vi "LV New.vi"(6 "Misc Project Files":path[](array[path]), 8 "error in (no error)":errorcluster, 9 "VI":path, 10 "Lvlib":path, 11 "Lvproj":path) -> (0 "error out":errorcluster)   [LabVIEW 2018, in "Pkg.lvlib"]
uses:
  Pkg.lvlib
  <vilib>/ErrorRing/Error Ring.xnode
  <vilib>/Utility/error.llb/Error Cluster From Error Code.vi
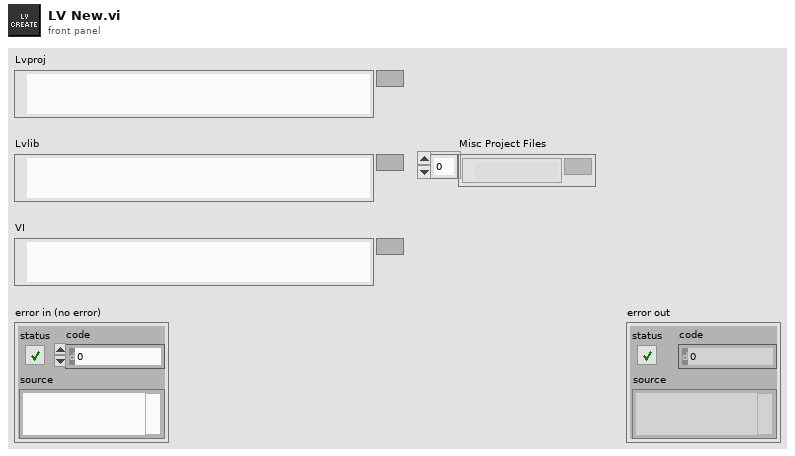
[diagram p1: front panel]
types:
  T1 = enum32{"invalid app kind", "Development System", "Run Time System", "Student Edition", "Embedded LabVIEW", "Evaluation", "Custom"}
  T2 = cluster{"Lvproj":path, "Lvlib":path, "VI":path, "RefLvproj":refnum<vi>, "RefLvlib":refnum<vi>, "RefVI":refnum<vi>, "IconText":string, "IconBG":u32, "MiscFiles":path[]}
  T3 = enum16{"Share clones between instances", "Preallocate clone for each instance"}
  T4 = typedef "imagedata.ctl" = cluster{"image type":i32, "image depth":i32, "image":u8[], "mask":u8[], "colors":u32[], "Rectangle":cluster{"left":i16, "top":i16, "right":i16, "bottom":i16}}
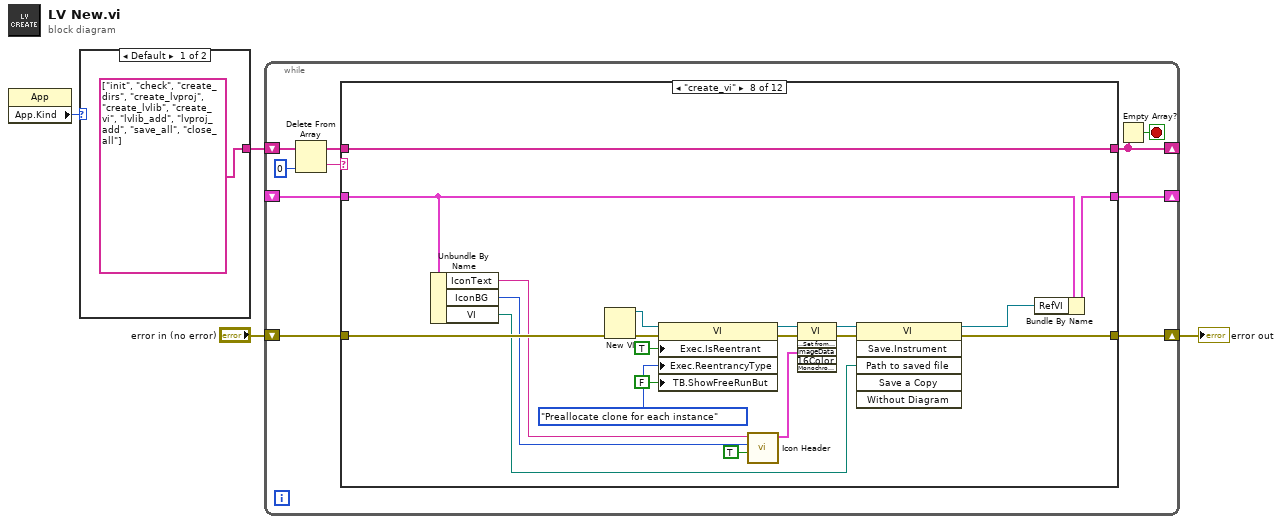
[diagram p0: block diagram]
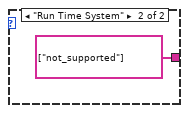
[diagram p2: hidden frame]
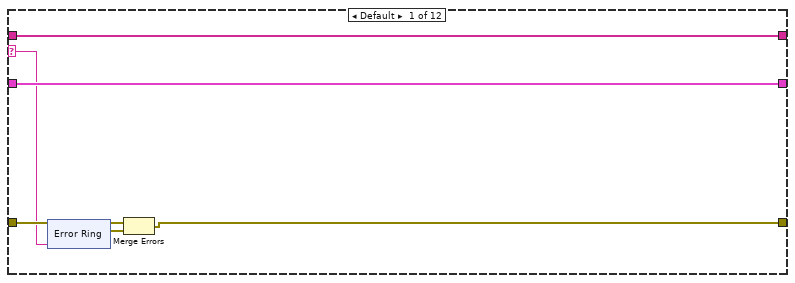
[diagram p3: hidden frame]
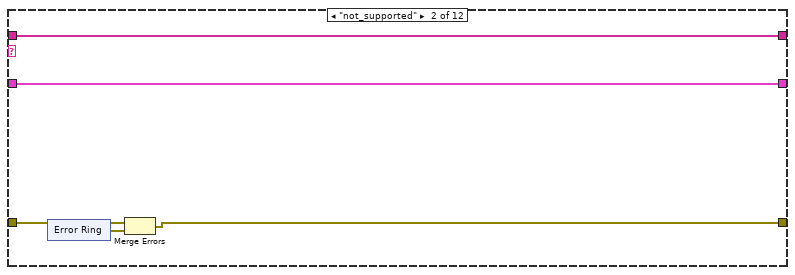
[diagram p4: hidden frame]
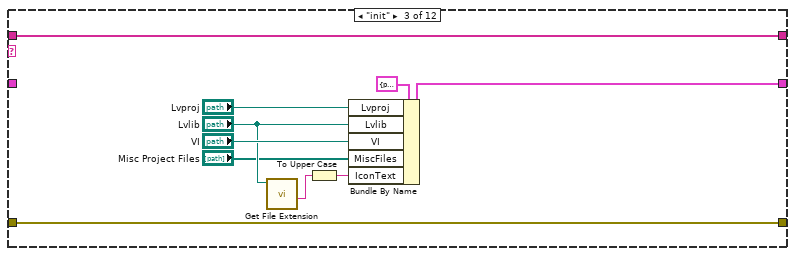
[diagram p5: hidden frame]
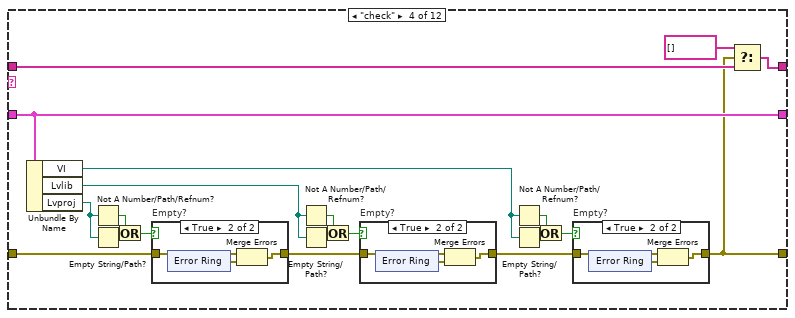
[diagram p6: hidden frame]
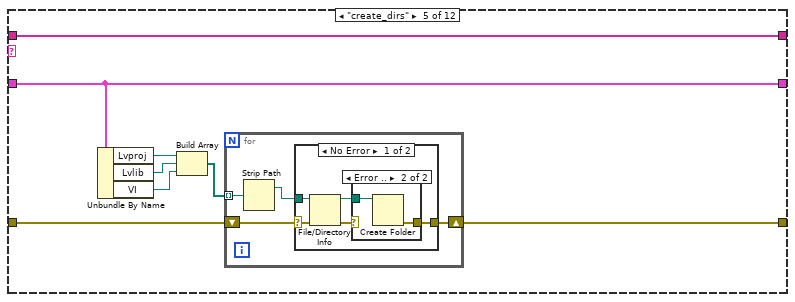
[diagram p10: hidden frame]
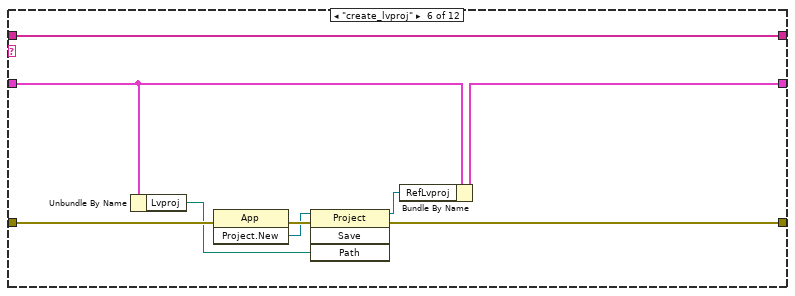
[diagram p13: hidden frame]
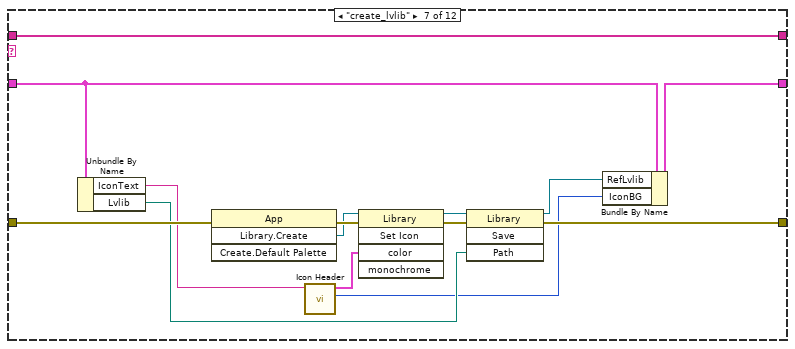
[diagram p14: hidden frame]
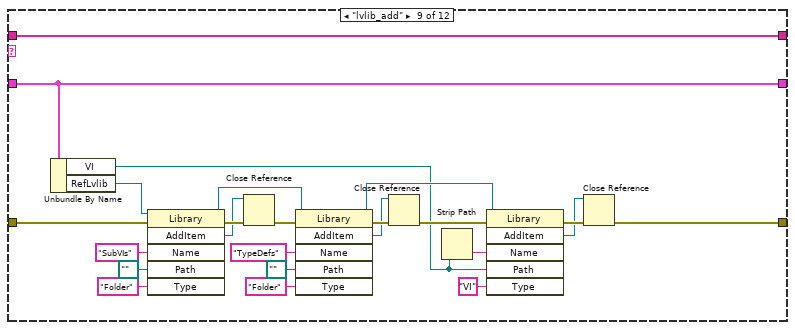
[diagram p15: hidden frame]
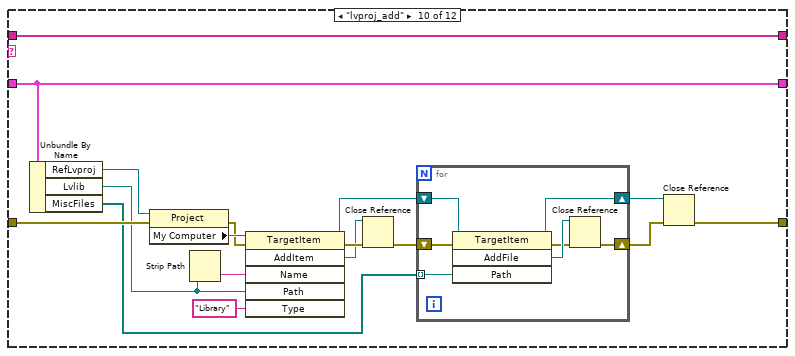
[diagram p16: hidden frame]
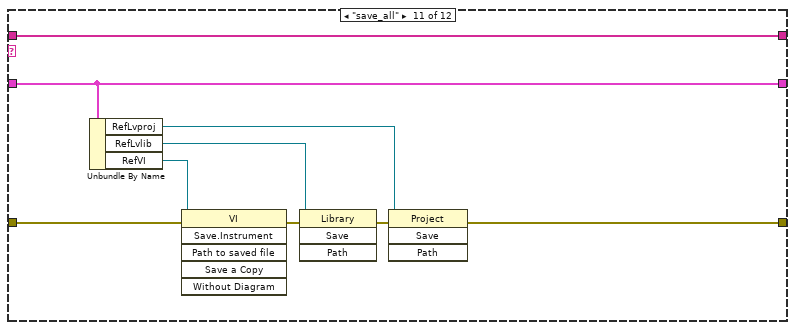
[diagram p17: hidden frame]
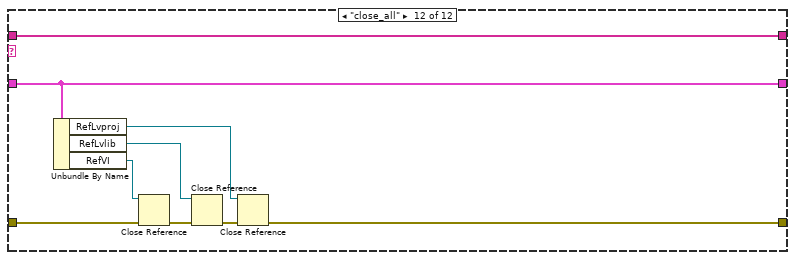
[diagram p18: hidden frame]
diagram:
  n1 = property class="App"() -> ("App.Kind"=w2:T1)  [unwired: 2 in, 2 out]
  n2 = case shown="Default" w2 {
    tunnel: [string[] ["init", "check", "create_dirs", "create_lvproj", "create_lvlib", "create_vi", "lvlib_add", "lvproj_add", "save_all", "close_all"] string[] ["not_supported"]] -> w1
    frame Default {
    }
    frame "Run Time System" {
    }
  }
  n3 = while {
    shift-right: [w12] -> _
    shift-left: w1 -> [w16]
    shift-right: [w8] -> _
    shift-left: _ -> [w7]
    shift-right: [w10] -> w3
    shift-left: "error in (no error)" -> [w9]
    stop <- w11 stop-if-true
    n4 = Delete From Array(array=w16, index=0) -> (deleted portion=w13:string, array with subset deleted=w15:string[])  [unwired: 1 in]
    n5 = case shown="\"create_vi\"" w13 {
      selector: w13 -> [w17 _ _ _ _ _ _ _ _ _ _ _]
      tunnel: w15 -> [w22 w34 w44 w69 w104 w126 w140 w160 w184 w201 w217 w226]
      tunnel: [w22 w34 w44 w52 w104 w126 w140 w160 w184 w201 w217 w226] -> w12
      tunnel: [w19 w31 w43 w51 w97 w122 w137 w156 w161 w190 w215 w224] -> w10
      tunnel: w9 -> [w21 w33 w43 w68 w103 w124 w138 w158 w164 w196 w216 w225]
      tunnel: [w20 w32 w48 w67 w102 w121 w136 w155 w183 w200 w214 w223] -> w8
      tunnel: w7 -> [w20 w32 _ w67 w102 w125 w139 w159 w183 w200 w214 w223]
      frame Default {
        n6 = xnode "Error Ring"("parameter 0"=w17) -> ("error out"=w18:errorcluster)
        n7 = Merge Errors(w21, w18) -> (w19:errorcluster)
      }
      frame "not_supported" {
        n8 = xnode "Error Ring"() -> ("error out"=w30:errorcluster)
        n9 = Merge Errors(w33, w30) -> (w31:errorcluster)
      }
      frame "init" {
        n10 = call <vilib>:"Get File Extension.vi"("file"="Lvlib") -> ("filename without extension"=w42:string)  [unwired: 6 in, 4 out]
        n11 = To Upper Case(1:w42) -> (0:w41:string)
        n12 = Bundle By Name(cluster=T2 {"Lvproj"=path "", "Lvlib"=path "", "VI"=path "", "RefLvproj"=refnum, "RefLvlib"=refnum, "RefVI"=refnum, "IconText"="", "IconBG"=0, "MiscFiles"=[]} ("StateData"), "Lvproj"="Lvproj", "Lvlib"="Lvlib", "VI"="VI", "MiscFiles"="Misc Project Files", "IconText"=w41) -> (w48:T2)
      }
      frame "check" {
        n13 = Unbundle By Name(w67) -> ("VI"=w53:path, "Lvlib"=w54:path, "Lvproj"=w64:path)
        n14 = Not A Number/Path/Refnum?(number/path/refnum=w64) -> (NaN/Path/Refnum?=w65:bool)
        n15 = Empty String/Path?(string/path=w64) -> (empty?=w66:bool)
        n16 = Or(x=w65, y=w66) -> (x .or. y?=w63:bool)
        n17 = case "Empty?" shown="True" w63 {
          tunnel: w68 -> [w88 w91]
          tunnel: [w88 w90] -> w55
          frame False {
          }
          frame True {
            n18 = xnode "Error Ring"() -> ("error out"=w89:errorcluster)
            n19 = Merge Errors(w91, w89) -> (w90:errorcluster)
          }
        }
        n20 = Not A Number/Path/Refnum?(number/path/refnum=w54) -> (NaN/Path/Refnum?=w61:bool)
        n21 = Empty String/Path?(string/path=w54) -> (empty?=w60:bool)
        n22 = Or(x=w61, y=w60) -> (x .or. y?=w62:bool)
        n23 = case "Empty?" shown="True" w62 {
          tunnel: w55 -> [w79 w82]
          tunnel: [w79 w81] -> w56
          frame False {
          }
          frame True {
            n24 = xnode "Error Ring"() -> ("error out"=w80:errorcluster)
            n25 = Merge Errors(w82, w80) -> (w81:errorcluster)
          }
        }
        n26 = Not A Number/Path/Refnum?(number/path/refnum=w53) -> (NaN/Path/Refnum?=w58:bool)
        n27 = Empty String/Path?(string/path=w53) -> (empty?=w59:bool)
        n28 = Or(x=w58, y=w59) -> (x .or. y?=w57:bool)
        n29 = case "Empty?" shown="True" w57 {
          tunnel: w56 -> [w70 w73]
          tunnel: [w70 w72] -> w51
          frame False {
          }
          frame True {
            n30 = xnode "Error Ring"() -> ("error out"=w71:errorcluster)
            n31 = Merge Errors(w73, w71) -> (w72:errorcluster)
          }
        }
        n32 = Select(t=string[] [], s=w51, f=w69) -> (s? t:f=w52:string[])
      }
      frame "create_dirs" {
        n33 = Unbundle By Name(w102) -> ("Lvproj"=w101:path, "Lvlib"=w100:path, "VI"=w99:path)
        n34 = Build Array(w101, w100, w99) -> (w98:path[])
        n35 = for {
          tunnel: w98 -> [w107] mode=indexing
          shift-right: [w106] -> w97
          shift-left: w103 -> [w108]
          n36 = Strip Path(path=w107) -> (stripped path=w105:path)  [unwired: 1 out]
          n37 = case shown="No Error" w108 {
            selector: w108 -> [w113 w117]
            tunnel: [w111 w117] -> w106
            tunnel: w105 -> [w109 _]
            frame No Error {
              n38 = File/Directory Info(path=w109, error in=w113) -> (path out=w110:path, error out=w112:errorcluster)  [unwired: 5 out]
              n39 = case shown="Error .." w112 {
                selector: w112 -> [w114 _]
                tunnel: [w114 w116] -> w111
                tunnel: w110 -> [_ w115]
                frame No Error {
                }
                frame Error {
                  n40 = Create Folder(path (use dialog)=w115) -> (error out=w116:errorcluster)  [unwired: 2 in, 2 out]
                }
              }
            }
            frame Error {
            }
          }
        }
      }
      frame "create_lvproj" {
        n41 = Unbundle By Name(w125) -> ("Lvproj"=w123:path)
        n42 = invoke class="App" method="Project.New"(error in=w124) -> (error out=w119:errorcluster, "Project:New"=w118:refnum<vi>)  [unwired: 2 in, 1 out]
        n43 = invoke class="Project" method="Save"(reference=w118, error in=w119, "Path"=w123) -> (reference out=w120:refnum<vi>, error out=w122:errorcluster)  [unwired: 1 in, 2 out]
        n44 = Bundle By Name(cluster=w125, "RefLvproj"=w120) -> (w121:T2)
      }
      frame "create_lvlib" {
        n45 = Unbundle By Name(w139) -> ("IconText"=w129:string, "Lvlib"=w128:path)
        n46 = invoke class="App" method="Library.Create"(error in=w138) -> (error out=w134:errorcluster, "Create Library"=w132:refnum<vi>)  [unwired: 3 in, 2 out]
        n47 = call "Icon Header.vi"("Text"=w129) -> ("BG out"=w127:u32, "Color256"=w130:T4)  [unwired: 9 in]
        n48 = invoke class="Library" method="Set Icon"(reference=w132, error in=w134, "color"=w130) -> (reference out=w131:refnum<vi>, error out=w133:errorcluster)  [unwired: 2 in, 3 out]
        n49 = invoke class="Library" method="Save"(reference=w131, error in=w133, "Path"=w128) -> (reference out=w135:refnum<vi>, error out=w137:errorcluster)  [unwired: 1 in, 2 out]
        n50 = Bundle By Name(cluster=w139, "RefLvlib"=w135, "IconBG"=w127) -> (w136:T2)
      }
      frame "create_vi" {
        n51 = Unbundle By Name(w159) -> ("IconText"=w153:string, "IconBG"=w142:u32, "VI"=w157:path)
        n52 = New VI(8:w158) -> (0:w152:errorcluster, 3:w150:refnum<vi>)  [unwired: 6 in]
        n53 = property class="VI"(reference=w150, error in=w152, "Exec.IsReentrant"=TRUE ("Execution:Is Reentrant"), "Exec.ReentrancyType"=T3."Preallocate clone for each instance" ("Execution:Reentrancy Type"), "TB.ShowFreeRunBut"=FALSE ("Tool Bar:Show Free Run Button")) -> (reference out=w146:refnum<vi>, error out=w151:errorcluster)
        n54 = call "Icon Header.vi"("Add Border? (F)"=TRUE, "BG (0=Random)"=w142, "Text"=w153) -> ("Color256"=w144:T4)  [unwired: 7 in, 1 out]
        n55 = invoke class="VI" method="VI Icon.Set from Image Data"(reference=w146, error in=w151, "ImageData"=w144) -> (reference out=w145:refnum<vi>, error out=w147:errorcluster)  [unwired: 3 in, 4 out]
        n56 = invoke class="VI" method="Save.Instrument"(reference=w145, error in=w147, "Path to saved file"=w157) -> (reference out=w154:refnum<vi>, error out=w156:errorcluster)  [unwired: 3 in, 4 out]
        n57 = Bundle By Name(cluster=w159, "RefVI"=w154) -> (w155:T2)
      }
      frame "lvlib_add" {
        n58 = Unbundle By Name(w183) -> ("VI"=w162:path, "RefLvlib"=w163:refnum<vi>)
        n59 = invoke class="Library" method="AddItem"(reference=w163, error in=w164, "Name"="SubVIs", "Path"=path "", "Type"="Folder") -> (reference out=w176:refnum<vi>, error out=w175:errorcluster, "AddItem"=w172:refnum<vi>)  [unwired: 1 in, 3 out]
        n60 = Close Reference(reference=w172, error in (no error)=w175) -> (error out=w173:errorcluster)
        n61 = invoke class="Library" method="AddItem"(reference=w176, error in=w173, "Name"="TypeDefs", "Path"=path "", "Type"="Folder") -> (reference out=w168:refnum<vi>, error out=w174:errorcluster, "AddItem"=w171:refnum<vi>)  [unwired: 1 in, 3 out]
        n62 = Close Reference(reference=w171, error in (no error)=w174) -> (error out=w165:errorcluster)
        n63 = Strip Path(path=w162) -> (name=w167:string)  [unwired: 1 out]
        n64 = invoke class="Library" method="AddItem"(reference=w168, error in=w165, "Name"=w167, "Path"=w162, "Type"="VI") -> (error out=w170:errorcluster, "AddItem"=w169:refnum<vi>)  [unwired: 1 in, 4 out]
        n65 = Close Reference(reference=w169, error in (no error)=w170) -> (error out=w161:errorcluster)
      }
      frame "lvproj_add" {
        n66 = Unbundle By Name(w200) -> ("RefLvproj"=w195:refnum<vi>, "Lvlib"=w192:path, "MiscFiles"=w185:path[])
        n67 = property class="Project"(reference=w195, error in=w196) -> (error out=w198:errorcluster, "My Computer"=w199:refnum<vi>)  [unwired: 1 out]
        n68 = Strip Path(path=w192) -> (name=w193:string)  [unwired: 1 out]
        n69 = invoke class="TargetItem" method="AddItem"(reference=w199, error in=w198, "Name"=w193, "Path"=w192, "Type"="Library") -> (reference out=w187:refnum<vi>, error out=w197:errorcluster, "AddItem"=w191:refnum<vi>)  [unwired: 1 in, 3 out]
        n70 = Close Reference(reference=w191, error in (no error)=w197) -> (error out=w189:errorcluster)
        n71 = for {
          shift-right: [w205] -> w188
          shift-left: w189 -> [w206]
          shift-right: [w203] -> w186
          shift-left: w187 -> [w204]
          tunnel: w185 -> [w202] mode=indexing
          n72 = invoke class="TargetItem" method="AddFile"(reference=w204, error in=w206, "Path"=w202) -> (reference out=w203:refnum<vi>, error out=w207:errorcluster, "AddFile"=w208:refnum<vi>)  [unwired: 1 in, 1 out]
          n73 = Close Reference(reference=w208, error in (no error)=w207) -> (error out=w205:errorcluster)
        }
        n74 = Close Reference(reference=w186, error in (no error)=w188) -> (error out=w190:errorcluster)
      }
      frame "save_all" {
        n75 = Unbundle By Name(w214) -> ("RefLvproj"=w211:refnum<vi>, "RefLvlib"=w212:refnum<vi>, "RefVI"=w213:refnum<vi>)
        n76 = invoke class="VI" method="Save.Instrument"(reference=w213, error in=w216) -> (error out=w210:errorcluster)  [unwired: 4 in, 5 out]
        n77 = invoke class="Library" method="Save"(reference=w212, error in=w210) -> (error out=w209:errorcluster)  [unwired: 2 in, 3 out]
        n78 = invoke class="Project" method="Save"(reference=w211, error in=w209) -> (error out=w215:errorcluster)  [unwired: 2 in, 3 out]
      }
      frame "close_all" {
        n79 = Unbundle By Name(w223) -> ("RefLvproj"=w220:refnum<vi>, "RefLvlib"=w221:refnum<vi>, "RefVI"=w222:refnum<vi>)
        n80 = Close Reference(reference=w222, error in (no error)=w225) -> (error out=w219:errorcluster)
        n81 = Close Reference(reference=w221, error in (no error)=w219) -> (error out=w218:errorcluster)
        n82 = Close Reference(reference=w220, error in (no error)=w218) -> (error out=w224:errorcluster)
      }
    }
    n83 = Empty Array?(array=w12) -> (empty?=w11:bool)
  }
  "error out" <- w3
